vi "TOML2JSON.vi"(8 "error in (no error)":errorcluster, 10 "Pretty Print? [F]":bool, 11 "toml_string":string="# This is a TOML document\n\ntitle = \"TOML Example\"\n\n[owner]\nname = \"Tom Preston-Werner\"\ndob = 1979-05-27T07:32:00-08:00\n\n[database]\nenabled = true\nports = [ 8000, 8001, 8002 ]\ndata = [ [\"delta\", \"phi\"], [3.14] ]\ntemp_targets = { cpu = 79.5, case = 72.0 }\n\n[servers]\n\n[servers.alpha]\nip = \"10.0.0.1\"\nrole = \"frontend\"\n\n[servers.beta]\nip = \"10.0.0.2\"\nrole = \"backend\"") -> (0 "error out":errorcluster, 3 "json_string":string)   [LabVIEW 2021, in "TOML2JSON.lvlib"]
uses:
  TOML2JSON.lvlib
  CLFN/cstring_free_memory.vi
  <vilib>/Utility/error.llb/Clear Errors.vi
  <vilib>/Utility/error.llb/Error Cluster From Error Code.vi
  <vilib>/ErrorRing/Error Ring.xnode
  include/TOML2JSON_64.dll
panel:
  out "json_string_len":u32
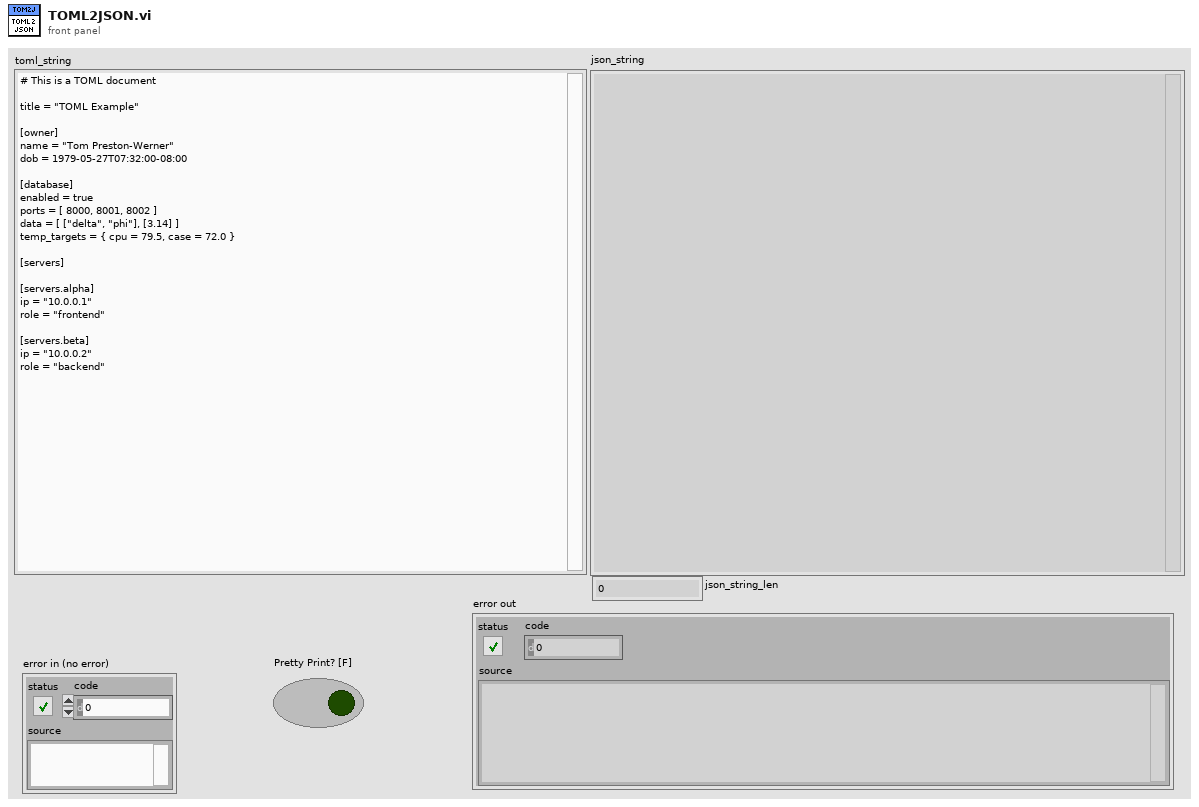
[diagram p1: front panel]
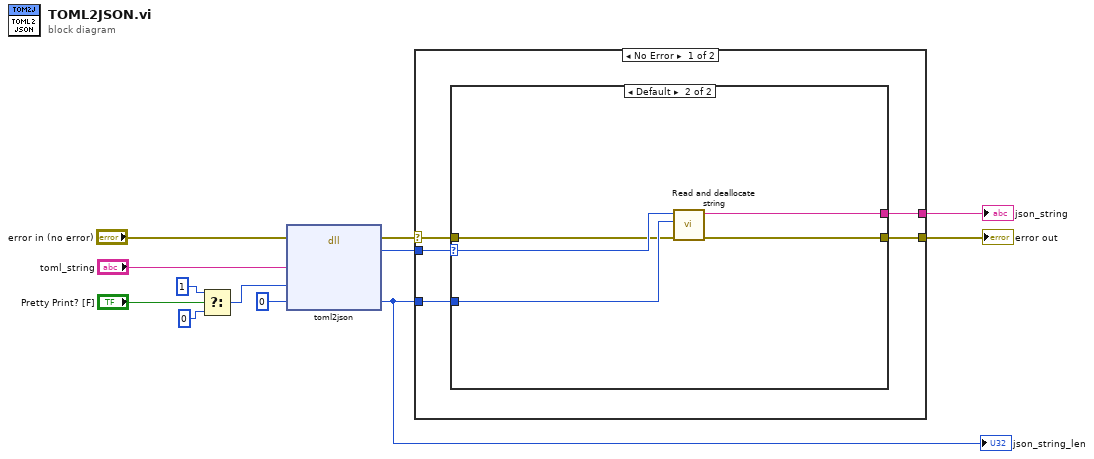
[diagram p0: block diagram]
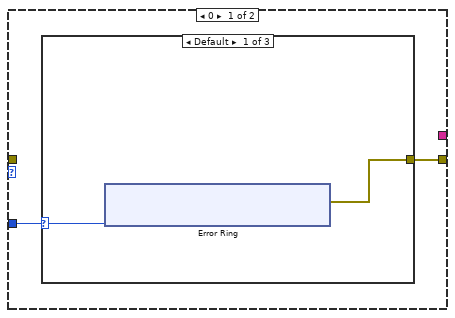
[diagram p2: hidden frame]
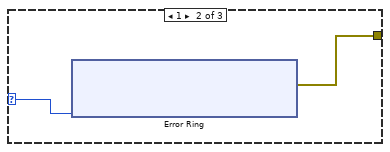
[diagram p3: hidden frame]
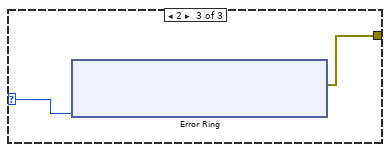
[diagram p4: hidden frame]
diagram:
  n1 = Select(t=u8 1 ("json_string_len"), s="Pretty Print? [F]", f=u8 0 ("prettyprint")) -> (s? t:f=w4:u8)
  n2 = dll-call lib="C:/GIT checkouts/LabVIEW-Kraken/Framework_Code/VIPs/TOML2JSON/lv_src/include/TOML2JSON_*.dll" fn="toml2json"(error in="error in (no error)", "toml_string"="toml_string", "prettyprint"=w4, "json_string_len"=u32 0) -> (error out=w2:errorcluster, "return type"=w3:u64, "json_string_len"=w1:u32)  [unwired: 4 in, 1 out]
  "json_string_len" <- w1
  n3 = case shown="No Error" w2 {
    selector: w2 -> [w14 w52]
    tunnel: [w13 w52] -> w10
    tunnel: [w17 _] -> w9
    tunnel: w1 -> [w16 _]
    tunnel: w3 -> [w15 _]
    frame No Error {
      n4 = case shown="Default" w15 {
        selector: w15 -> [_ w49]
        tunnel: [_ w51] -> w17
        tunnel: w16 -> [w19 w50]
        tunnel: w14 -> [_ w48]
        tunnel: [w18 w47] -> w13
        frame 0 {
          n5 = case shown="Default" w19 {
            selector: w19 -> [w21 w30 w39]
            tunnel: [w20 w29 w38] -> w18
            frame Default {
              n6 = xnode "Error Ring"("parameter 0"=w21) -> ("error out"=w20:errorcluster)
            }
            frame 1 {
              n7 = xnode "Error Ring"("parameter 0"=w30) -> ("error out"=w29:errorcluster)
            }
            frame 2 {
              n8 = xnode "Error Ring"("parameter 0"=w39) -> ("error out"=w38:errorcluster)
            }
          }
        }
        frame Default {
          n9 = call "Read and deallocate string.vi"("error in (no error)"=w48, "string_len"=w50, "string_ptr"=w49) -> ("error out"=w47:errorcluster, "string"=w51:string)  [unwired: 7 in]
        }
      }
    }
    frame Error {
    }
  }
  "error out" <- w10
  "json_string" <- w9
